vi "Actor Core.vi"(8 "error in":errorcluster, 11 "Study Actor in":refnum<class "Study Actor.lvclass">) -> (0 "error out":errorcluster, 3 "Actor out":refnum<class "Actor.lvclass">)   [LabVIEW 2023, in "Study Actor.lvlib" / "Study Actor.lvclass"]
doc: "The user interface for this panel.\n\n----\nPlease see the following web address for additional documentation and tutorial information:\nhttp://www.mooregoodideas.com/mgi-panel-manager/\n\nAuthor: Derek Trepanier\n\nCopyright (c) 2018, Moore Good Ideas, Inc.\n\nAll rights reserved.\n\nRedistribution and use in source and binary forms, with or without modification, are permitted provided that the following conditions are met:\n\n * Redistributions of source code must retain the above copyright notice, this list of conditions and the following disclaimer.\n * Redistributions in binary form must reproduce the above copyright notice, this list of conditions and the following disclaimer in the documentation and/or other materials provided with the distribution.\n * Neither the name of Moore Good Ideas, Inc. nor the names of its contributors may be used to endorse or promote products derived from this software without specific prior written permission.\n\nTHIS SOFTWARE IS PROVIDED BY THE COPYRIGHT HOLDERS AND CONTRIBUTORS \"AS IS\" AND ANY EXPRESS OR IMPLIED WARRANTIES, INCLUDING, BUT NOT LIMITED TO, THE IMPLIED WARRANTIES OF MERCHANTABILITY AND FITNESS FOR A PARTICULAR PURPOSE ARE DISCLAIMED. IN NO EVENT SHALL THE COPYRIGHT OWNER OR CONTRIBUTORS BE LIABLE FOR ANY DIRECT, INDIRECT, INCIDENTAL, SPECIAL, EXEMPLARY, OR CONSEQUENTIAL DAMAGES (INCLUDING, BUT NOT LIMITED TO, PROCUREMENT OF SUBSTITUTE GOODS OR SERVICES; LOSS OF USE, DATA, OR PROFITS; OR BUSINESS INTERRUPTION) HOWEVER CAUSED AND ON ANY THEORY OF LIABILITY, WHETHER IN CONTRACT, STRICT LIABILITY, OR TORT (INCLUDING NEGLIGENCE OR OTHERWISE) ARISING IN ANY WAY OUT OF THE USE OF THIS SOFTWARE, EVEN IF ADVISED OF THE POSSIBILITY OF SUCH DAMAGE."
uses:
  Study Actor.lvclass
  <vilib>/ActorFramework/Actor/Actor.lvclass
  DIO/DIO DAQmx Simulated CFGs/DO DAQmx PWM Fixed Freq CFG/DO DAQmx Fixed Freq PWM CFG.lvclass
  DIO/Virtual DIO/Virt PWM Fixed Freq Generator/Virt DAQmx Fixed Freq PWM Generator.lvclass
  Tests/Sample Series/Sample PWM Fans/Sample PWM Fans/Sample PWM Fans.lvclass
  DIO/DO DAQmx Fixed Freq PWM CFG/DO DAQmx Fixed Freq PWM CFG.lvclass
  Study Actor.lvclass/Study Actor.ctl
  <vilib>/ActorFramework/Message Enqueuer/Message Enqueuer.lvclass/Message Enqueuer.ctl
  IStudy Actor Messages/Launch Series Msg/Launch Series Msg.lvclass/Launch Series Msg.ctl
  <vilib>/ActorFramework/Message Enqueuer/Enqueue.vi
  <vilib>/ActorFramework/Stop Msg/Stop Msg.lvclass
  IStudy Actor Messages/Launch Series Msg/Launch Series Msg.lvclass
  <vilib>/Utility/LVClass/Get LV Class Name.vi
  <resource>/AFDebug/Generate Trace for Message.vi
  <vilib>/ActorFramework/Message Priority Queue/Priority Enqueue.vi
  <vilib>/MGI/Panel Manager/Panel Actor/Panel Actor/Panel Actor.lvclass
panel:
  in  "Series CFG":string="{\n    \"Name\": \"Fan Test Series\",\n    \"Series Actor Class\": \"Sample PWM Fans.lvlib:Sample PWM Fans.lvclass\",\n    \"GUID\": \"\",\n    \"Instr CFGs\": [],\n    \"Virt Instrs\": [],\n    \"Tasks\": [\n        {\n            \"Ident\": \"Stack1\",\n            \"Class\": \"Sample PWM Fan.lvclass\",\n            \"Point Idents\": [\n                \"Fan1\"\n            ]\n        },\n        {\n            \"Ident\": \"Stack2\",\n            \"Class\": \"Sample PWM Fan.lvclass\",\n            \"Point Idents\": [\n                \"Fan2\"\n            ]\n        }\n    ]\n}"
  in  "Virt Instrs":string="{\n    \"Virt Instrs\": [\n        {\n            \"Point Ident\": \"Fan1\",\n            \"Instr Ident\": \"DIO9403\",\n            \"Const Action Data\": \"port0/line0\",\n            \"Class\": \"Virt Instrs DIO.lvlib:Virt DAQmx Fixed Freq PWM Generator.lvclass\"\n        },\n        {\n            \"Point Ident\": \"Fan2\",\n            \"Instr Ident\": \"DIO9403\",\n            \"Const Action Data\": \"port0/line2\",\n            \"Class\": \"Virt Instrs DIO.lvlib:Virt DAQmx Fixed Freq PWM Generator.lvclass\"\n        }\n    ]\n}"
  in  "Instr CFGs":string[](array[string])
  in  "Launch Series Button":bool
  out "Connected":bool
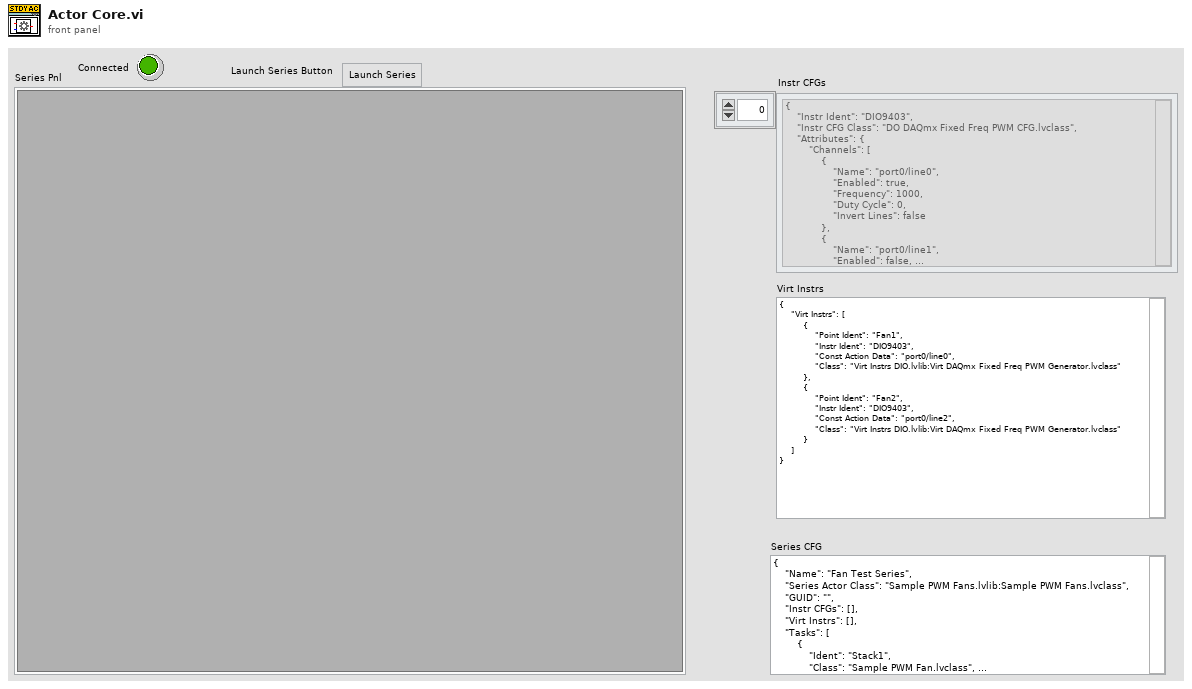
[diagram p1: front panel]
types:
  T1 = cluster{"Pnl Actor":refnum<event-registration>, "Event Registration Refnum":refnum<event-registration>}
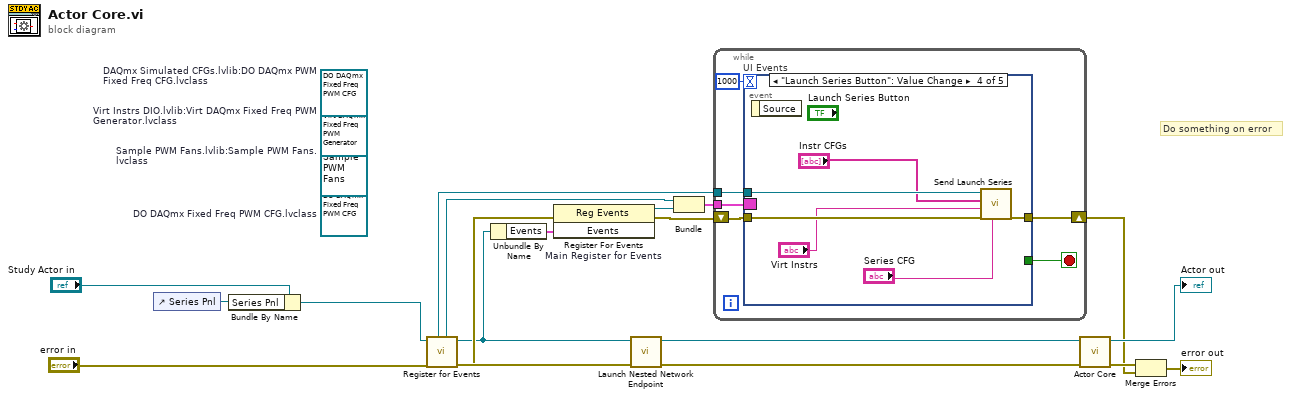
[diagram p0: block diagram]
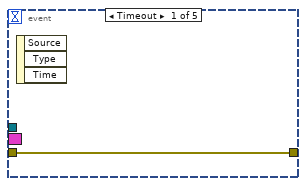
[diagram p2: hidden frame]
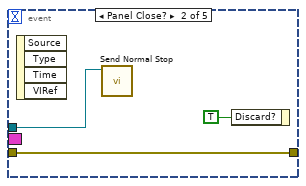
[diagram p3: hidden frame]
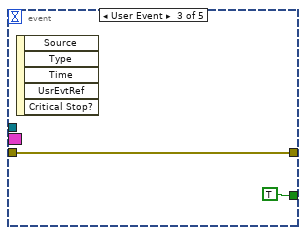
[diagram p4: hidden frame]
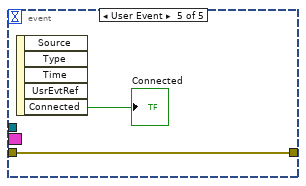
[diagram p5: hidden frame]
diagram:
  (unwired) refnum<class "DO DAQmx Fixed Freq PWM CFG.lvclass"> refnum  # DO DAQmx Fixed Freq PWM CFG.lvclass
  (unwired) refnum<class "Sample PWM Fans.lvclass"> refnum  # Sample PWM Fans.lvlib:Sample PWM Fans.lvclass
  (unwired) refnum<class "Virt DAQmx Fixed Freq PWM Generator.lvclass"> refnum  # Virt Instrs DIO.lvlib:Virt DAQmx Fixed Freq PWM Generator.lvclass
  (unwired) refnum<class "DO DAQmx Fixed Freq PWM CFG.lvclass"> refnum  # DAQmx Simulated CFGs.lvlib:DO DAQmx PWM Fixed Freq CFG.lvclass
  # "Do something on error"
  n1 = control-ref of="Series Pnl"() -> (w15:refnum<vi>)
  n2 = Bundle By Name(cluster="Study Actor in", "Series Pnl"=w15) -> (w13:refnum<class "Study Actor.lvclass">)
  n3 = call <vilib>:"Register for Events.vi"("Error In"="error in", "Panel Actor in"=w13) -> ("Error Out"=w9:errorcluster, "Panel Actor out"=w1:refnum<class "Study Actor.lvclass">, "Pnl Actor"=w8:refnum<event-registration>, "Self Enqueuer"=w7:refnum<class "Message Enqueuer.lvclass">)  [unwired: 6 in]
  n4 = Unbundle By Name(w1) -> ("Events"=w10:cluster{"Connected":refnum<user-event>})
  n5 = call "Launch Nested Network Endpoint.vi"("error in"=w9, "Study Actor in"=w1) -> ("error out"=w3:errorcluster, "Study Actor out"=w2:refnum<class "Study Actor.lvclass">)  [unwired: 8 in]
  n6 = register-events "Main Register for Events"(error in=w3, w10) -> (reference out=w12:refnum<event-registration>, error out=w6:errorcluster)  [unwired: 1 in]
  n7 = Bundle("Pnl Actor"=w8, "Event Registration Refnum"=w12) -> (w11:T1)  [unwired: 1 in]
  n8 = while {
    tunnel: w11 -> [w24]
    tunnel: w7 -> [w23]
    shift-right: [w19] -> w4
    shift-left: w6 -> [w22]
    stop <- w20 stop-if-true
    n9 = event "UI Events" shown="[3] \"Launch Series Button\": Value Change" {
      selector: w24 -> [_ _ _ _ _]
      dyn-events: _ -> [_ _ _ _ _]
      timeout: 1000 -> [_ _ _ _ _]
      tunnel: [_ _ TRUE _ _] -> w20
      tunnel: w23 -> [_ w28 _ w36 _]
      tunnel: w22 -> [w25 w26 w29 w35 w37]
      tunnel: [w25 w26 w29 w34 w37] -> w19
      event Timeout {
        n10 = event-data() -> ()  [unwired: 1 in, 3 out]
      }
      event Panel Close? {
        n11 = event-data() -> ()  [unwired: 1 in, 4 out]
        n12 = call <vilib>:"Send Normal Stop.vi"("Message Enqueuer"=w28) -> ()  [unwired: 10 in, 1 out]
        n13 = event-data("Discard?"=TRUE) -> ()  [unwired: 1 in, 1 out]
      }
      event User Event {
        n14 = event-data() -> ()  [unwired: 1 in, 5 out]
      }
      event "Launch Series Button": Value Change {
        n15 = event-data() -> ()  [unwired: 1 in, 1 out]
        n16 = call "Send Launch Series.vi"("Series CFG"="Series CFG", "error in (no error)"=w35, "Virt Instrs"="Virt Instrs", "Instr CFGs"="Instr CFGs", "Message Enqueuer"=w36) -> ("error out"=w34:errorcluster)  [unwired: 5 in, 1 out]
      }
      event User Event {
        n17 = event-data() -> ("Connected"=→"Connected":bool)  [unwired: 1 in, 4 out]
      }
    }
  }
  n18 = call-parent "Actor Core.vi"("error in"=w3, "Panel Actor in"=w2) -> ("error out"=w18:errorcluster, "Actor out"=→"Actor out":refnum<class "Actor.lvclass">)  [unwired: 8 in]
  n19 = Merge Errors(w18, w4) -> (→"error out":errorcluster)
